vi "保存报表-电子表格.vi"(9 "测试数据":string, 11 "保存报表信息簇":T1) -> ()   [LabVIEW 2011]
panel:
  out "appended path":path
  out "dup path":path
  out "添加的路径":path
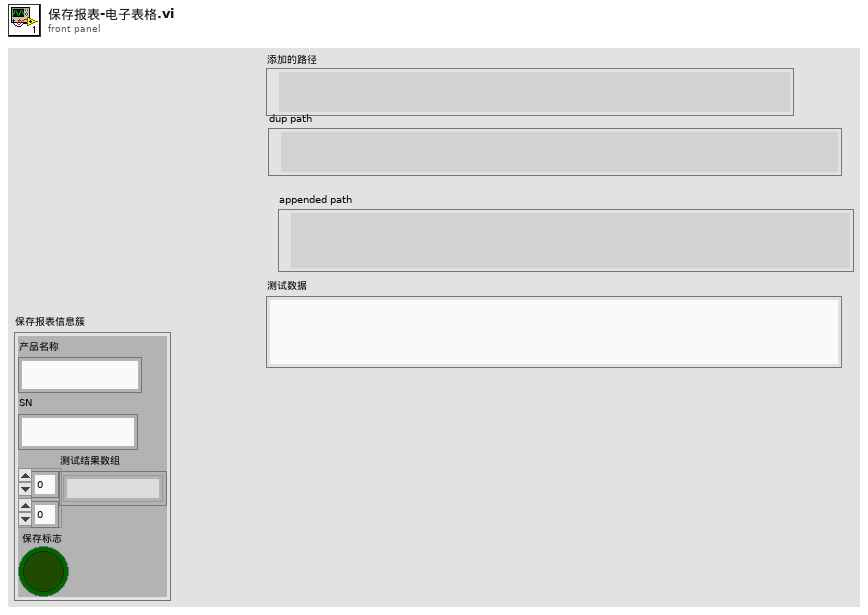
[diagram p1: front panel]
types:
  T1 = cluster{"产品名称":string, "SN":string, "测试结果数组":string[][], "保存标志":bool}
  T2 = enum16{"open", "replace", "create", "open or create", "replace or create", "replace or create with confirmation"}
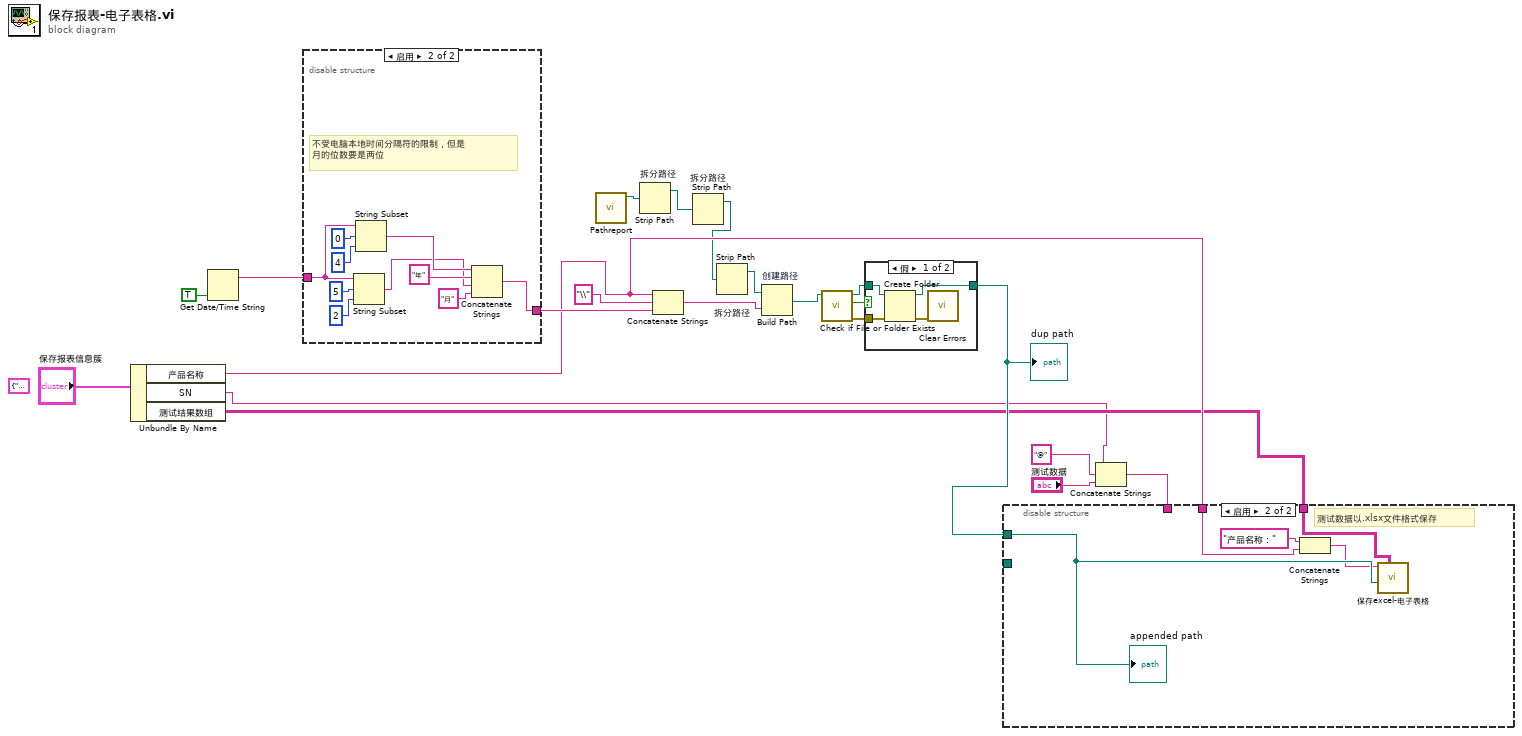
[diagram p0: block diagram]
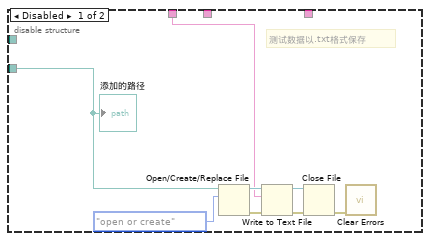
[diagram p2: hidden frame]
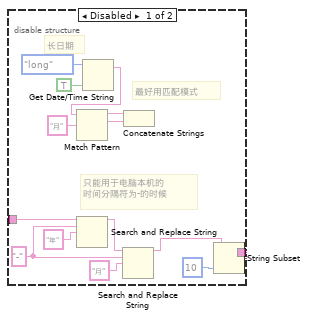
[diagram p3: hidden frame]
diagram:
  (unwired) T1 {"产品名称"="", "SN"="", "测试结果数组"=[], "保存标志"=FALSE} ("保存报表信息簇")
  n1 = Unbundle By Name("保存报表信息簇") -> ("产品名称"=w8:string, "SN"=w1:string, "测试结果数组"=w7:string[][])
  n2 = Get Date/Time String(want seconds? (F)=TRUE ("需要秒？(F)")) -> (date string=w16:string)  [unwired: 2 in, 1 out]
  n3 = disable-structure shown="启用" {
    disable-tunnel: [w29 w36] -> w14
    disable-tunnel: w16 -> [w28 w41]
    frame Disabled {
      w34 = "-" ("搜索字符串")
      # "长日期"
      # "最好用匹配模式"
      # "只能用于电脑本机的\n时间分隔符为-的时候"
      n4 = Search and Replace String(input string=w28, search string=w34, replace string="年" ("替换字符串(\"\")")) -> (result string=w30:string)  [unwired: 5 in, 3 out]
      n5 = Get Date/Time String(date format (0)=enum16{"short", "long", "abbreviated"}."long" ("日期格式(0)"), want seconds? (F)=TRUE ("需要秒？(F)")) -> (date string=w24:string)  [unwired: 1 in, 1 out]
      n6 = Match Pattern(string=w24, regular expression="月" ("正则表达式")) -> (before substring=w23:string, match substring=w22:string)  [unwired: 1 in, 2 out]
      n7 = Search and Replace String(input string=w30, search string=w34, replace string="月" ("替换字符串(\"\")")) -> (result string=w32:string)  [unwired: 5 in, 3 out]
      n8 = Concatenate Strings(w23, w22) -> ()  [unwired: 1 out]
      n9 = String Subset(string=w32, length (rest)=10 ("长度（剩余）")) -> (substring=w29:string)  [unwired: 1 in]
    }
    frame Enabled {
      # "不受电脑本地时间分隔符的限制，但是\n月的位数要是两位"
      n10 = String Subset(string=w41, offset (0)=5 ("偏移量(0)"), length (rest)=2 ("长度（剩余）")) -> (substring=w38:string)
      n11 = String Subset(string=w41, offset (0)=0 ("偏移量(0)"), length (rest)=4 ("长度（剩余）")) -> (substring=w40:string)
      n12 = Concatenate Strings(w40, "年" ("替换字符串(\"\")"), w38, "月" ("替换字符串(\"\")")) -> (w36:string)
    }
  }
  n13 = call "Pathreport.vi"() -> ("appended path"=w19:path)  [unwired: 11 in]
  n14 = Strip Path "拆分路径"(path=w19) -> (stripped path=w5:path)  [unwired: 1 out]
  n15 = Concatenate Strings(w8, "\\" ("搜索字符串"), w14) -> (w2:string)
  n16 = Strip Path "拆分路径"(path=w5) -> (stripped path=w4:path)  [unwired: 1 out]
  n17 = Strip Path "拆分路径"(path=w4) -> (stripped path=w3:path)  [unwired: 1 out]
  n18 = Build Path "创建路径"(base path=w3, name or relative path=w2) -> (appended path=w6:path)
  n19 = call <vilib>:"Check if File or Folder Exists.vi"("path"=w6) -> ("error out"=w17:errorcluster, "file or folder exists?"=w21:bool, "dup path"=w20:path)  [unwired: 8 in]
  n20 = case shown="假" w21 {
    tunnel: w20 -> [w48 w50]
    tunnel: [w49 w50] -> w10
    tunnel: w17 -> [w47 _]
    frame False {
      n21 = Create Folder(path (use dialog)=w48, error in=w47) -> (created path=w49:path, error out=w46:errorcluster)  [unwired: 1 in, 1 out]
      n22 = call <vilib>:"Clear Errors.vi"("error in (no error)"=w46) -> ()  [unwired: 6 in, 1 out]
    }
    frame True {
    }
  }
  "dup path" <- w10
  n23 = Concatenate Strings(w1, "@" ("字符串"), "测试数据") -> (w11:string)
  n24 = disable-structure shown="启用" {
    disable-tunnel: w8 -> [_ w62]
    disable-tunnel: w11 -> [w52 _]
    disable-tunnel: w7 -> [_ w61]
    disable-tunnel: _ -> [w51 _]
    disable-tunnel: w10 -> [_ w60]
    frame Disabled {
      # "测试数据以.txt格式保存"
      n25 = Open/Create/Replace File(file path (use dialog)=w51, operation (0:open)=T2."open or create" ("操作(0:open)")) -> (refnum out=w57:refnum<file>, error out=w56:errorcluster)  [unwired: 4 in, 1 out]
      n26 = Write to Text File(file (use dialog)=w57, text=w52, error in=w56) -> (refnum out=w54:refnum<file>, error out=w55:errorcluster)  [unwired: 1 in, 1 out]
      n27 = Close File(refnum=w54, error in=w55) -> (error out=w53:errorcluster)  [unwired: 1 out]
      n28 = call <vilib>:"Clear Errors.vi"("error in (no error)"=w53) -> ()  [unwired: 6 in, 1 out]
      "添加的路径" <- w51
    }
    frame Enabled {
      # "测试数据以.xlsx文件格式保存"
      n29 = Concatenate Strings("产品名称：" ("字符串"), w62) -> (w59:string)
      n30 = call "保存excel-电子表格.vi"("测试数据"=w61, "保存路径"=w60, "标题"=w59) -> ()  [unwired: 9 in]
      "appended path" <- w60
    }
  }
